vi "build_state_frame.vi"(8 "error in":errorcluster, 11 "State sensor sample":string) -> (0 "error out":errorcluster, 3 "New State Frame":string)   [LabVIEW 2019]
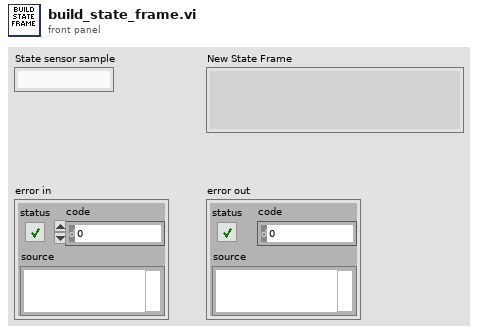
[diagram p1: front panel]
types:
  T1 = cluster{"frame":cluster{"vehicles":cluster{"state":cluster{"color":string, "name":string, "odometry":cluster{"angular_velocity":cluster{"x":dbl, "y":dbl, "z":dbl}, "linear_velocity":cluster{"x":dbl, "y":dbl, "z":dbl}, "pose":cluster{"orientation":cluster{"w":dbl, "x":dbl, "y":dbl, "z":dbl}, "position":cluster{"x":dbl, "y":dbl, "z":dbl}}}, "replay_class":string, "tags":string[]}, "wheels":cluster{"id":i32, "pose":cluster{"orientation":cluster{"w":dbl, "x":dbl, "y":dbl, "z":dbl}, "position":cluster{"x":dbl, "y":dbl, "z":dbl}}, "speed":dbl}[]}[]}, "game_time":dbl, "sample_count":dbl, "time":dbl}
  T2 = cluster{"state_frame":cluster{"frame":cluster{"vehicles":cluster{"state":cluster{"color":string, "name":string, "odometry":cluster{"angular_velocity":cluster{"x":dbl, "y":dbl, "z":dbl}, "linear_velocity":cluster{"x":dbl, "y":dbl, "z":dbl}, "pose":cluster{"orientation":cluster{"w":dbl, "x":dbl, "y":dbl, "z":dbl}, "position":cluster{"x":dbl, "y":dbl, "z":dbl}}}, "replay_class":string, "tags":string[]}, "wheels":cluster{"id":i32, "pose":cluster{"orientation":cluster{"w":dbl, "x":dbl, "y":dbl, "z":dbl}, "position":cluster{"x":dbl, "y":dbl, "z":dbl}}, "speed":dbl}[]}[]}, "game_time":dbl, "sample_count":dbl, "time":dbl}, "time_step":dbl}
  T3 = cluster{"state":cluster{"color":string, "name":string, "odometry":cluster{"angular_velocity":cluster{"x":dbl, "y":dbl, "z":dbl}, "linear_velocity":cluster{"x":dbl, "y":dbl, "z":dbl}, "pose":cluster{"orientation":cluster{"w":dbl, "x":dbl, "y":dbl, "z":dbl}, "position":cluster{"x":dbl, "y":dbl, "z":dbl}}}, "replay_class":string, "tags":string[]}, "wheels":cluster{"id":i32, "pose":cluster{"orientation":cluster{"w":dbl, "x":dbl, "y":dbl, "z":dbl}, "position":cluster{"x":dbl, "y":dbl, "z":dbl}}, "speed":dbl}[]}[]
  T4 = cluster{"state":cluster{"color":string, "name":string, "odometry":cluster{"angular_velocity":cluster{"x":dbl, "y":dbl, "z":dbl}, "linear_velocity":cluster{"x":dbl, "y":dbl, "z":dbl}, "pose":cluster{"orientation":cluster{"w":dbl, "x":dbl, "y":dbl, "z":dbl}, "position":cluster{"x":dbl, "y":dbl, "z":dbl}}}, "replay_class":string, "tags":string[]}, "wheels":cluster{"id":i32, "pose":cluster{"orientation":cluster{"w":dbl, "x":dbl, "y":dbl, "z":dbl}, "position":cluster{"x":dbl, "y":dbl, "z":dbl}}, "speed":dbl}[]}
  T5 = cluster{cluster{"state":cluster{"color":string, "name":string, "odometry":cluster{"angular_velocity":cluster{"x":dbl, "y":dbl, "z":dbl}, "linear_velocity":cluster{"x":dbl, "y":dbl, "z":dbl}, "pose":cluster{"orientation":cluster{"w":dbl, "x":dbl, "y":dbl, "z":dbl}, "position":cluster{"x":dbl, "y":dbl, "z":dbl}}}, "replay_class":string, "tags":string[]}, "wheels":cluster{"id":i32, "pose":cluster{"orientation":cluster{"w":dbl, "x":dbl, "y":dbl, "z":dbl}, "position":cluster{"x":dbl, "y":dbl, "z":dbl}}, "speed":dbl}[]}[]}
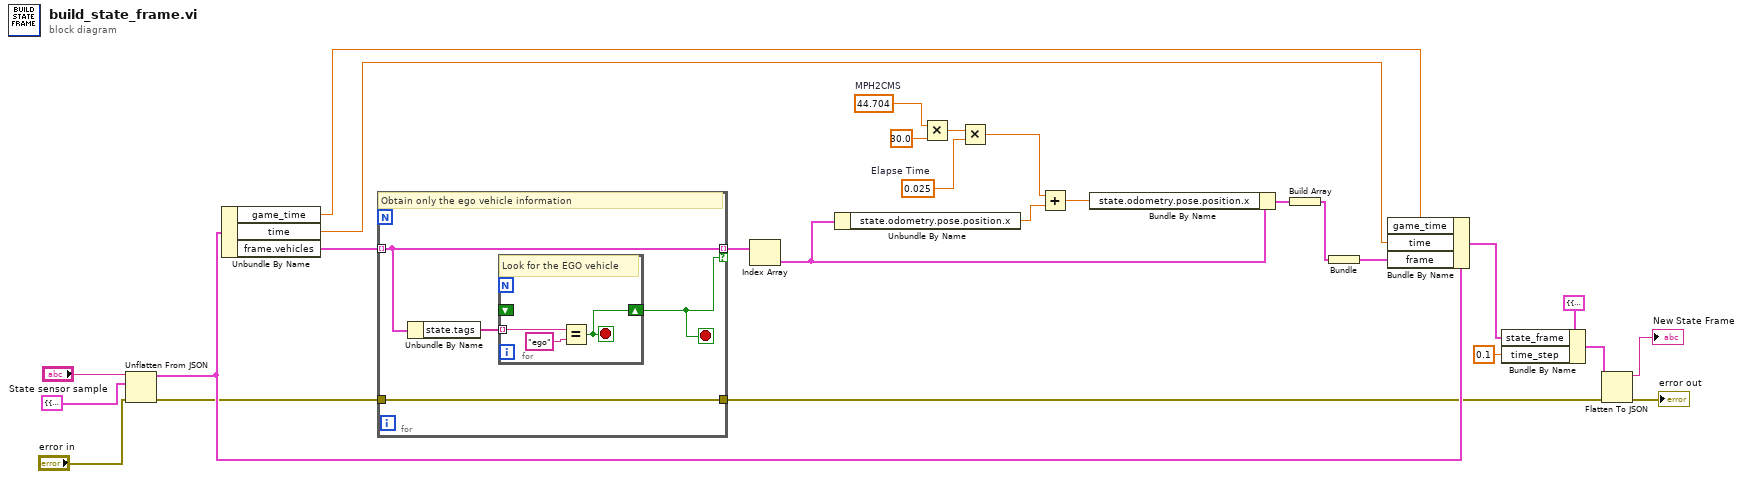
[diagram p0: block diagram]
diagram:
  w6 = 0.025  # Elapse Time
  w9 = 44.704  # MPH2CMS
  n1 = Unflatten From JSON(JSON string="State sensor sample", type and defaults=T1 {"frame"={"vehicles"=[]}, "game_time"=0.0, "sample_count"=0.0, "time"=0.0} ("Cluster"), error in (no error)="error in") -> (value=w27:T1, error out=w14:errorcluster)  [unwired: 4 in]
  n2 = Unbundle By Name(w27) -> ("game_time"=w2:dbl, "time"=w1:dbl, "frame.vehicles"=w18:T3)
  n3 = for {
    tunnel: w18 -> [w29] mode=indexing
    tunnel: [w29] -> w13 mode=indexing if=w28
    tunnel: w14 -> [w30]
    tunnel: [w30] -> w16
    stop <- w28 stop-if-true
    # "Obtain only the ego vehicle information"
    n4 = Unbundle By Name(w29) -> ("state.tags"=w31:string[])
    n5 = for {
      tunnel: w31 -> [w34] mode=indexing
      shift-right: [w32] -> w28
      shift-left: _ -> [_]
      stop <- w32 stop-if-true
      # "Look for the EGO vehicle"
      n6 = Equal?(x=w34, y="ego") -> (x = y?=w32:bool)
    }
  }
  n7 = Index Array(array=w13) -> (element=w12:T4)  [unwired: 1 in]
  n8 = Unbundle By Name(w12) -> ("state.odometry.pose.position.x"=w4:dbl)
  n9 = Multiply(x=w9, y=30.0) -> (x*y=w7:dbl)
  n10 = Multiply(x=w7, y=w6) -> (x*y=w3:dbl)
  n11 = Add(x=w3, y=w4) -> (x+y=w5:dbl)
  n12 = Bundle By Name(cluster=w12, "state.odometry.pose.position.x"=w5) -> (w11:T4)
  n13 = Build Array(w11) -> (w10:T3)
  n14 = Bundle(w10) -> (w20:T5)  [unwired: 1 in]
  n15 = Bundle By Name(cluster=w27, "game_time"=w2, "time"=w1, "frame"=w20) -> (w24:T1)
  n16 = Bundle By Name(cluster=T2 {"state_frame"={"frame"={"vehicles"=[]}, "game_time"=0.0, "sample_count"=0.0, "time"=0.0}, "time_step"=0.0} ("Cluster"), "state_frame"=w24, "time_step"=0.1) -> (w21:T2)
  n17 = Flatten To JSON(anything=w21, error in (no error)=w16) -> (JSON string=→"New State Frame":string, 11:→"error out":errorcluster)  [unwired: 1 in]
